vi "BK Precision 91xx (GPIB) RT Driver VI.vi"(6 "Device Clock":string, 9 "Device Inputs FIFO":refnum<k33>, 10 "Device Outputs FIFO":refnum<k33>, 11 "Device Reference":T1 format="%.0x") -> ()   [LabVIEW 2011, in "BK Precision 91xx (GPIB) Custom Device.lvlib"]
uses:
  BK Precision 91xx (GPIB) Custom Device.lvlib
  <vilib>/NI Veristand/Custom Device API/Custom Device Item Ref.ctl
  <vilib>/NI Veristand/Custom Device API/Custom Device Channel Type.ctl
  <vilib>/Platform/TimedLoop/XDataNode/timing_clust.ctl
  <vilib>/Platform/TimedLoop/XDataNode/nitl_modes.ctl
  <vilib>/Platform/TimedLoop/XDataNode/wakeup.ctl
  <vilib>/Platform/TimedLoop/XDataNode/XDataNode.xnode
  <vilib>/Platform/TimedLoop/XDataNode/XDNodeRunTimeDep.lvlib
  <vilib>/NI Veristand/Custom Device API/Custom Device API.lvlib
  <vilib>/NI Veristand/Custom Device Tools/Custom Device Utility Library/Custom Device Utility Library.lvlib
panel:
  in  "Status Notifier":refnum<notifier>
  # "Custom Device Template\nv1.0"
  # "Use this template as a starting point for creating a custom device code module. The input controls shown here are specially named controls that the system will use to provide the device loop with data. The controls are not required for the device loop to run. For instance, if the device doesn't produce any output data, then you don't need the Device Outputs FIFO control. If you do use these controls, however, they need to have these exact names to be functional."
  # "The optional status notifier element is used to notify the RT engine of the last state of the custom device, and to indicate the device has completed execution. If this control is not used, a default No Error value is returned to the system when the device finishes execution.\n\nNote: This error state is not checked until the system shuts down. Use an output status channel to send more immediate status values to the system."
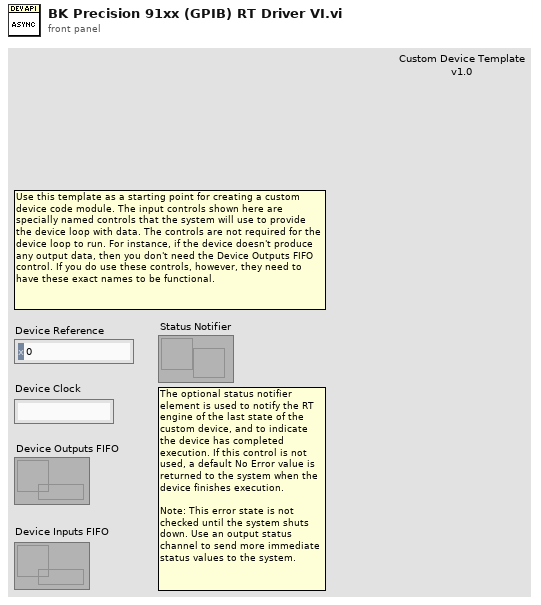
[diagram p1: front panel]
types:
  T1 = typedef "Custom Device API.lvlib/Custom Device Item Ref.ctl" = u64
  T2 = typedef "Custom Device API.lvlib/Custom Device Channel Type.ctl" = enum16{"Input", "Output"}
  T3 = typedef "BK Precision 91xx (GPIB) Custom Device.lvlib/Serial Config.ctl" = cluster{"Baud Rate":u32, "Parity":u16, "Data Bits":u16, "Stop Bits":u16}
  T4 = typedef "Custom Device API.lvlib/Custom Device Timed Loop Priority.ctl" = enum32{"Low", "Medium", "High"}
  T5 = typedef "XDNodeRunTimeDep.lvlib/timing_clust.ctl" = cluster{"Expected End [f-1]":u64, "Actual End [f-1]":u64, "Finished Late? [f-1]":bool, "Expected End [i-1]":u64, "Actual End [i-1]":u64, "Finished Late? [i-1]":bool, "Expected Start [i]":u64, "Actual Start [i]":u64, "Expected Start [f]":u64, "Actual Start [f]":u64, "Source Name":string, "Structure Name":string, "Period":i64, "Deadline":i64, "Offset":i64, "Start":i64, "Priority":i32, "Timeout":i32, "Mode":T6, "Wakeup Reason":T7, "Error":errorcluster, "Source Type":string, "Secondary Source Type":string, "Global End Time":u64, "Global Start Time":u64, "Frame Duration":u64, "Iteration Duration":u64, "Assigned CPU":i32, "I/O Scan Engine Mode":u32}
  T6 = typedef "XDNodeRunTimeDep.lvlib/nitl_modes.ctl" = enum32{"No Change", "Process missed periods, maintain original phase", "Discard missed periods, maintain original phase", "Process missed periods, ignore original phase", "Discard missed periods, ignore original phase"}
  T7 = typedef "XDNodeRunTimeDep.lvlib/wakeup.ctl" = enum32{"Normal", "Aborted", "Asynchronous wakeup", "Timing source error", "Timed loop error", "Timeout"}
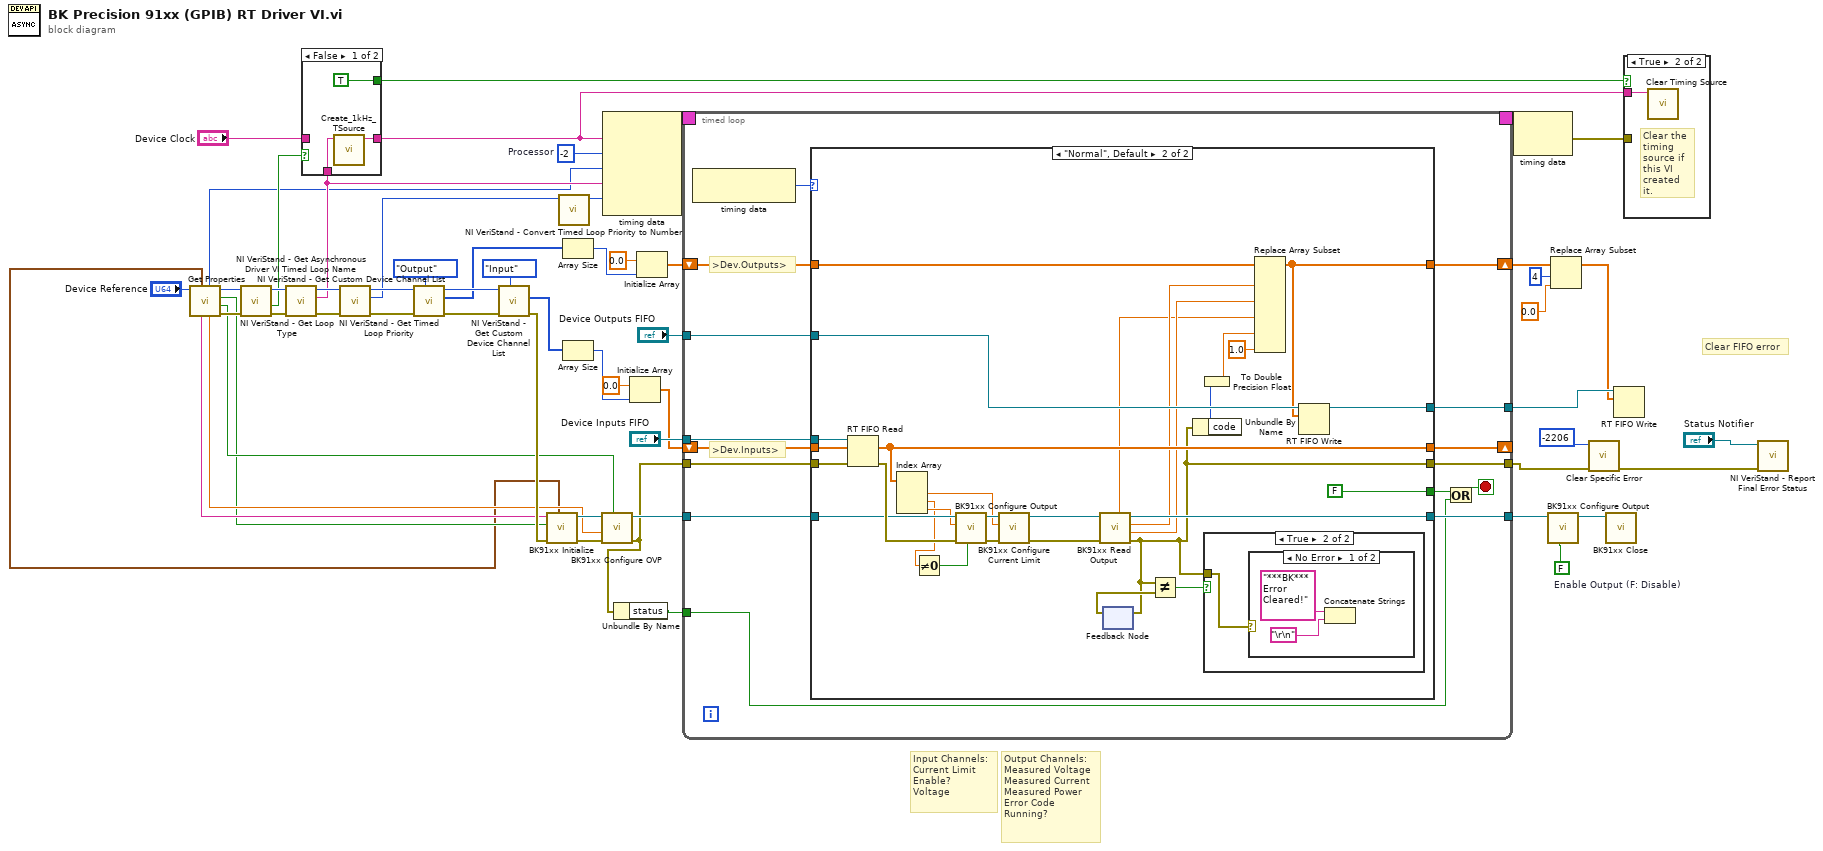
[diagram p0: block diagram]
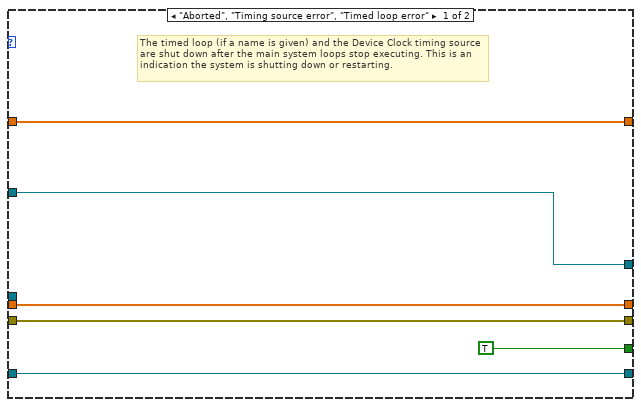
[diagram p4: hidden frame]
diagram:
  w16 = FALSE items=["OFF", "ON", "OFF", "ON"]  # Enable Output (F: Disable)
  w38 = -2  # Processor
  # "Clear FIFO error"
  # "Output Channels:\nMeasured Voltage\nMeasured Current\nMeasured Power\nError Code\nRunning?"
  # "Input Channels:\nCurrent Limit\nEnable?\nVoltage"
  n1 = call "Get Properties.vi"("Device Reference In"="Device Reference") -> ("error out"=w26:errorcluster, "Enable OVP"=w20:bool, "ID Query?"=w13:bool, "Device Reference Out"=w24:T1, "Voltage Limit"=w21:dbl, "Update Rate"=w18:u16, "VISA Resource Name"=w22:string, "serial"=w1:T3)  [unwired: 3 in]
  n2 = call <vilib>:"NI VeriStand - Get Loop Type.vi"("error in (no error)"=w26, "Device Ref in"=w24) -> ("error out"=w36:errorcluster, "Use Device Clock"=w34:bool, "Device Ref out"=w35:T1)  [unwired: 7 out]
  n3 = call <vilib>:"NI VeriStand - Get Asynchronous Driver VI Timed Loop Name.vi"("error in (no error)"=w36, "Device Ref in"=w35) -> ("error out"=w42:errorcluster, "Device Timed Loop Name"=w29:string, "Device Ref out"=w58:T1)  [unwired: 7 out]
  n4 = case shown="False" w34 {
    tunnel: "Device Clock" -> [_ w62]
    tunnel: [w61 w62] -> w14
    tunnel: [TRUE _] -> w30
    tunnel: w29 -> [w59 _]
    frame False {
      n5 = call <vilib>:"Create_1kHz_TSource.vi"("name (in)"=w59) -> ("name (out)"=w61:string)  [unwired: 1 in, 9 out]
    }
    frame True {
    }
  }
  n6 = call <vilib>:"NI VeriStand - Get Timed Loop Priority.vi"("error in (no error)"=w42, "Device Ref in"=w58) -> ("error out"=w43:errorcluster, "Priority"=w40:T4, "Device Ref out"=w44:T1)  [unwired: 7 out]
  n7 = call <vilib>:"NI VeriStand - Get Custom Device Channel List.vi"("Channel Type"=Custom_Device_Channel_Type."Output", "error in (no error)"=w43, "Device Ref in"=w44) -> ("error out"=w47:errorcluster, "Specified Channel Ref List"=w12:T1[], "Device Ref out"=w48:T1)  [unwired: 6 out]
  n8 = call <vilib>:"NI VeriStand - Get Custom Device Channel List.vi"("Channel Type"=Custom_Device_Channel_Type."Input", "error in (no error)"=w47, "Device Ref in"=w48) -> ("error out"=w23:errorcluster, "Specified Channel Ref List"=w41:T1[])  [unwired: 7 out]
  n9 = call "BK91xx Initialize.vi"("Serial Configuration"=w1, "error in (no error)"=w23, "ID Query (True)"=w13, "VISA resource name"=w22) -> ("error out"=w28:errorcluster, "VISA resource name out"=w27:refnum<visa-resource-name>)  [unwired: 6 in]
  n10 = call <vilib>:"NI VeriStand - Convert Timed Loop Priority to Number.vi"("Priority"=w40) -> ("Numeric Priority"=w39:i32)  [unwired: 10 out]
  n11 = Array Size(array=w12) -> (size(s)=w45:i32)
  n12 = Array Size(array=w41) -> (size(s)=w37:i32)
  n13 = call "BK91xx Configure OVP.vi"("Enable OVP (T: Enable)"=w20, "error in (no error)"=w28, "Voltage Limit (20.000000 V)"=w21, "VISA resource name"=w27) -> ("error out"=w8:errorcluster, "VISA resource name out"=w19:refnum<visa-resource-name>)  [unwired: 6 in]
  n14 = node-c288(w14, w38, w18, w29, w39) -> (w55:T5)
  n15 = Unbundle By Name(w8) -> ("status"=w7:bool)
  n16 = Initialize Array(0.0 ("element"), w37) -> (w50:dbl[])
  n17 = Initialize Array(0.0 ("element"), w45) -> (w51:dbl[])
  n18 = timed-loop {
    timing: w55 -> [_]
    timing-out: [_] -> w54
    shift-right: [w75] -> _
    shift-left: w50 -> [w76]
    shift-right: [w72] -> w5
    shift-left: w51 -> [w73]
    tunnel: "Device Outputs FIFO" -> [w71]
    tunnel: "Device Inputs FIFO" -> [w70]
    tunnel: w19 -> [w69]
    tunnel: [w68] -> w15
    tunnel: w8 -> [w77]
    tunnel: [w66] -> w11
    tunnel: w7 -> [w64]
    tunnel: [w63] -> w6
    stop <- w65 stop-if-true
    # ">Dev.Outputs>"
    # ">Dev.Inputs>"
    n19 = node-c288() -> (w74:T7)  [unwired: 1 out]
    n20 = case shown="\"Normal\", Default" w74 {
      tunnel: w77 -> [w82 w107]
      tunnel: w76 -> [w83 w109]
      tunnel: [w82 w84] -> w66
      tunnel: [w83 w106] -> w75
      tunnel: w73 -> [w81 w110]
      tunnel: [w81 w108] -> w72
      tunnel: w71 -> [w78 w112]
      tunnel: w70 -> [_ w111]
      tunnel: [TRUE FALSE] -> w67
      tunnel: w69 -> [w79 w104]
      tunnel: [w79 w101] -> w68
      tunnel: [w78 w87] -> w63
      frame "Aborted", "Timing source error", "Timed loop error" {
        # "The timed loop (if a name is given) and the Device Clock timing source are shut down after the main system loops stop executing. This is an indication the system is shutting down or restarting."
      }
      frame "Normal", Default {
        n21 = RT FIFO Read(0:w111, 1:w109, 3:w107) -> (9:w106:dbl[], 11:w105:errorcluster)  [unwired: 4 out]
        n22 = Index Array(array=w106) -> (element #1=w99:dbl, element #2=w96:dbl, element #3=w98:dbl)  [unwired: 3 in]
        n23 = Not Equal To 0?(x=w96) -> (x != 0?=w97:bool)
        n24 = call "BK91xx Configure Output.vi"("Enable Output (T: Enable)"=w97, "error in (no error)"=w105, "Voltage Level (0.000000 V)"=w98, "VISA resource name"=w104) -> ("error out"=w103:errorcluster, "VISA resource name out"=w102:refnum<visa-resource-name>)  [unwired: 6 in]
        n25 = call "BK91xx Configure Current Limit.vi"("error in (no error)"=w103, "Current Limit (0.000000 A)"=w99, "VISA resource name"=w102) -> ("error out"=w90:errorcluster, "VISA resource name out"=w89:refnum<visa-resource-name>)  [unwired: 7 in]
        n26 = call "BK91xx Read Output.vi"("error in (no error)"=w90, "VISA resource name"=w89) -> ("error out"=w84:errorcluster, "Measured Current Level (A)"=w94:dbl, "Measured Voltage Level (V)"=w95:dbl, "VISA resource name out"=w101:refnum<visa-resource-name>, "Measured Power Level (W)"=w91:dbl)  [unwired: 5 in]
        n27 = feedback-in #1(w84) -> ()
        n28 = feedback #1() -> (w86:errorcluster)  [unwired: 1 in]
        n29 = Not Equal?(x=w84, y=w86) -> (x != y?=w85:bool)
        n30 = Unbundle By Name(w84) -> ("code"=w93:i32)
        n31 = To Double Precision Float(number=w93) -> (double precision float=w92:dbl)
        n32 = case shown="True" w85 {
          tunnel: w84 -> [_ w113]
          frame False {
          }
          frame True {
            n33 = case shown="No Error" w113 {
              frame No Error {
                n34 = Concatenate Strings("***BK*** Error Cleared!" ("string"), "\r\n") -> ()  [unwired: 1 out]
              }
              frame Error {
              }
            }
          }
        }
        n35 = Replace Array Subset(array=w110, new element #1=w95, new element #2=w94, new element #3=w91, new element #4=w92, new element #5=1.0 ("new element/subarray")) -> (w108:dbl[])  [unwired: 5 in]
        n36 = RT FIFO Write(0:w112, 1:w108) -> (8:w87:refnum<k33>)  [unwired: 2 in, 4 out]
      }
    }
    n37 = Or(x=w67, y=w64) -> (x .or. y?=w65:bool)
  }
  n38 = node-c288(w54) -> (w31:errorcluster)
  n39 = call "BK91xx Configure Output.vi"("Enable Output (T: Enable)"=w16, "VISA resource name"=w15) -> ("VISA resource name out"=w17:refnum<visa-resource-name>)  [unwired: 8 in, 1 out]
  n40 = Replace Array Subset(array=w5, new element=0.0 ("new element/subarray"), index=4) -> (w4:dbl[])
  n41 = call "Clear Specific Error.vi"("error in (no error)"=w11, "code"=-2206 ("x")) -> ("error out"=w9:errorcluster)  [unwired: 9 in]
  n42 = call "BK91xx Close.vi"("VISA resource name"=w17) -> ()  [unwired: 10 in, 1 out]
  n43 = RT FIFO Write(0:w6, 1:w4) -> ()  [unwired: 2 in, 5 out]
  n44 = case shown="True" w30 {
    tunnel: w31 -> [_ _]
    tunnel: w14 -> [_ w119]
    frame False {
    }
    frame True {
      # "Clear the timing source if this VI created it."
      n45 = call <vilib>:"Clear Timing Source.vi"("name"=w119) -> ()  [unwired: 1 in, 10 out]
    }
  }
  n46 = call <vilib>:"NI VeriStand - Report Final Error Status.vi"("error in (no error)"=w9, "Status Notifier"="Status Notifier") -> ()  [unwired: 1 in, 9 out]
